vi "Evaluate Expression.vi"(8 "Part In":map{string, i64}(c390), 11 "Expression":string) -> (1 "Pass/Fail":bool)   [LabVIEW 2021]
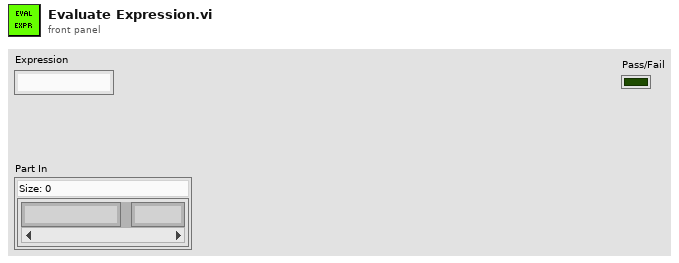
[diagram p1: front panel]
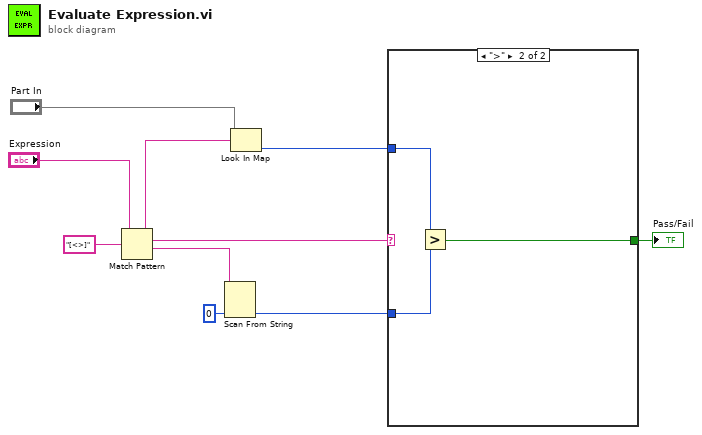
[diagram p0: block diagram]
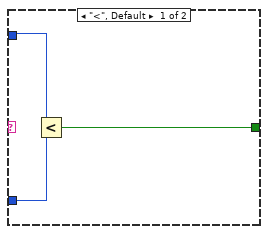
[diagram p2: hidden frame]
diagram:
  n1 = Match Pattern(string="Expression", regular expression="[<>]") -> (before substring=w7:string, match substring=w8:string, after substring=w4:string)  [unwired: 1 in, 1 out]
  n2 = Scan From String(input string=w4, default 1=i64 0) -> (output 1=w2:i64)  [unwired: 3 in, 3 out]
  n3 = Look In Map(map="Part In", key=w7) -> (value=w5:i64)  [unwired: 1 in, 1 out]
  n4 = case shown="\">\"" w8 {
    tunnel: w5 -> [w12 w15]
    tunnel: w2 -> [w13 w14]
    tunnel: [w11 w16] -> w1
    frame "<", Default {
      n5 = Less?(x=w12, y=w13) -> (x < y?=w11:bool)
    }
    frame ">" {
      n6 = Greater?(x=w15, y=w14) -> (0:w16:bool)
    }
  }
  "Pass/Fail" <- w1
